vi "health_initVars.vi"(11 "hDin":T1={"nSignals"=0, "logname"="", "time"=timestamp(0 s since 1904-01-01), "dir"=path "", "adamSerial"={"port"="COM1", "timeout"=1000, "baud"=9600, "dataBits"=8, "stopBits"=10, "flowControl"=0, "parity"=0, "termChar"=FALSE, "checkSum"=FALSE}, "fiberSerial"={"port1"="COM1", "port2"="COM1", "timeout"=1000, "baud"=9600, "dataBits"=8, "stopBits"=10, "flowControl"=0, "parity"=0, "termChar"=FALSE, "checkSum"=FALSE, "fiber1On"=FALSE, "fiber2On"=FALSE}, "signal"={"src"=[], "id"=[], "ch"=[], "descrip"=[], "units"=[], "scale"=[], "hi"=[], "lo"=[], "rec"=[], "fault"=[], "val"=[]}, "teSerial"={"port"="COM1", "timeout"=1000, "baud"=9600, "dataBits"=8, "stopBits"=10, "flowControl"=0, "parity"=0, "termChar"=FALSE, "checkSum"=FALSE, "checkSumVal"=""}, "lograte"=0, "calSwitch"=FALSE, "logoffset"=0.0} {"teSerial"."stopBits" items=["1.0"=10, "1.5"=15, "2.0"=20]; "teSerial"."parity" items=["None", "Odd", "Even", "Mark", "Space"]; "teSerial"."flowControl" items=["None"=0, "XON/XOFF"=1, "RTS/CTS"=2, "DTR/DSR"=4]; "fiberSerial"."stopBits" items=["1.0"=10, "1.5"=15, "2.0"=20]; "fiberSerial"."parity" items=["None", "Odd", "Even", "Mark", "Space"]; "fiberSerial"."flowControl" items=["None"=0, "XON/XOFF"=1, "RTS/CTS"=2, "DTR/DSR"=4]; "adamSerial"."stopBits" items=["1.0"=10, "1.5"=15, "2.0"=20]; "adamSerial"."parity" items=["None", "Odd", "Even", "Mark", "Space"]; "adamSerial"."flowControl" items=["None"=0, "XON/XOFF"=1, "RTS/CTS"=2, "DTR/DSR"=4]}) -> (3 "hDout":T1={"nSignals"=0, "logname"="", "time"=timestamp(0 s since 1904-01-01), "dir"=path "", "adamSerial"={"port"="COM1", "timeout"=1000, "baud"=9600, "dataBits"=8, "stopBits"=10, "flowControl"=0, "parity"=0, "termChar"=FALSE, "checkSum"=FALSE}, "fiberSerial"={"port1"="COM1", "port2"="COM1", "timeout"=1000, "baud"=9600, "dataBits"=8, "stopBits"=10, "flowControl"=0, "parity"=0, "termChar"=FALSE, "checkSum"=FALSE, "fiber1On"=FALSE, "fiber2On"=FALSE}, "signal"={"src"=[], "id"=[], "ch"=[], "descrip"=[], "units"=[], "scale"=[], "hi"=[], "lo"=[], "rec"=[], "fault"=[], "val"=[]}, "teSerial"={"port"="COM1", "timeout"=1000, "baud"=9600, "dataBits"=8, "stopBits"=10, "flowControl"=0, "parity"=0, "termChar"=FALSE, "checkSum"=FALSE, "checkSumVal"=""}, "lograte"=0, "calSwitch"=FALSE, "logoffset"=0.0} {"teSerial"."stopBits" items=["1.0"=10, "1.5"=15, "2.0"=20]; "teSerial"."parity" items=["None", "Odd", "Even", "Mark", "Space"]; "teSerial"."flowControl" items=["None"=0, "XON/XOFF"=1, "RTS/CTS"=2, "DTR/DSR"=4]; "fiberSerial"."stopBits" items=["1.0"=10, "1.5"=15, "2.0"=20]; "fiberSerial"."parity" items=["None", "Odd", "Even", "Mark", "Space"]; "fiberSerial"."flowControl" items=["None"=0, "XON/XOFF"=1, "RTS/CTS"=2, "DTR/DSR"=4]; "adamSerial"."stopBits" items=["1.0"=10, "1.5"=15, "2.0"=20]; "adamSerial"."parity" items=["None", "Odd", "Even", "Mark", "Space"]; "adamSerial"."flowControl" items=["None"=0, "XON/XOFF"=1, "RTS/CTS"=2, "DTR/DSR"=4]})   [LabVIEW 2018]
uses:
  health_Loop_Clust.ctl
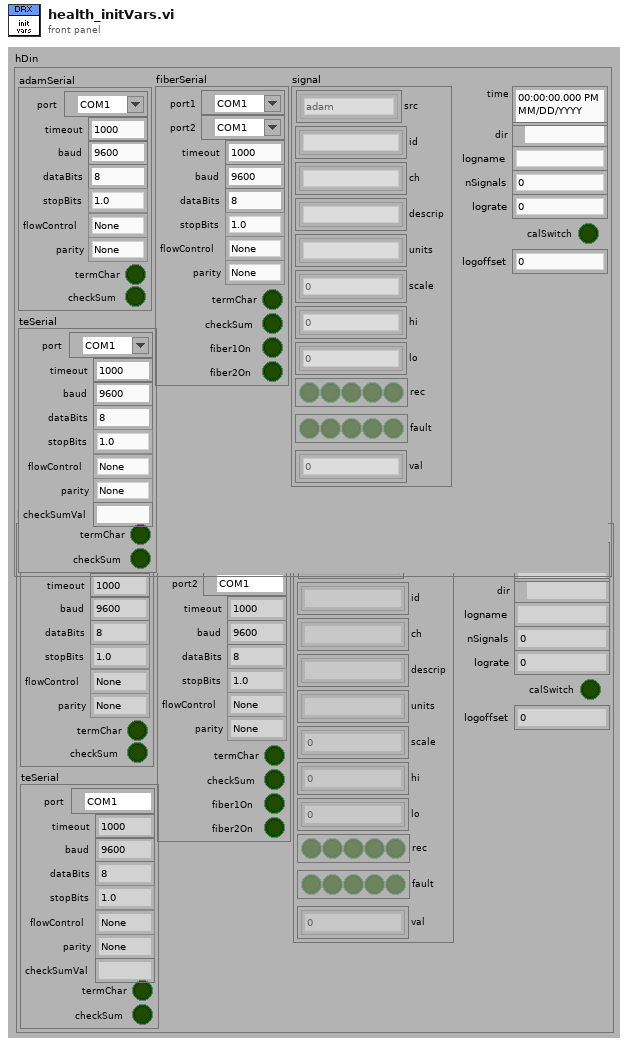
[diagram p1: front panel]
types:
  T1 = typedef "health_Loop_Clust.ctl" = cluster{"nSignals":i32, "logname":string, "time":timestamp, "dir":path, "adamSerial":cluster{"port":refnum<visa-resource-name>, "timeout":u32, "baud":u32, "dataBits":u16, "stopBits":u16, "flowControl":u16, "parity":u16, "termChar":bool, "checkSum":bool}, "fiberSerial":cluster{"port1":refnum<visa-resource-name>, "port2":refnum<visa-resource-name>, "timeout":u32, "baud":u32, "dataBits":u16, "stopBits":u16, "flowControl":u16, "parity":u16, "termChar":bool, "checkSum":bool, "fiber1On":bool, "fiber2On":bool}, "signal":cluster{"src":enum16{"adam", "fiber", "te"}[], "id":string[], "ch":string[], "descrip":string[], "units":string[], "scale":dbl[], "hi":dbl[], "lo":dbl[], "rec":bool[], "fault":bool[], "val":dbl[]}, "teSerial":cluster{"port":refnum<visa-resource-name>, "timeout":u32, "baud":u32, "dataBits":u16, "stopBits":u16, "flowControl":u16, "parity":u16, "termChar":bool, "checkSum":bool, "checkSumVal":string}, "lograte":u32, "calSwitch":bool, "logoffset":dbl}
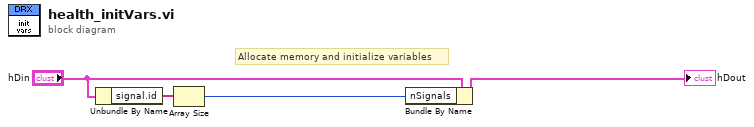
[diagram p0: block diagram]
diagram:
  # "Allocate memory and initialize variables"
  n1 = Unbundle By Name("hDin") -> ("signal.id"=w4:string[])
  n2 = Array Size(array=w4) -> (size(s)=w2:i32)
  n3 = Bundle By Name(cluster="hDin", "nSignals"=w2) -> (→"hDout":T1)
